vi "TEMPLATE_Constructor.vi"(8 "Error In":errorcluster) -> (0 "Error Out":errorcluster, 3 "OpaqueStruct Out":refnum<class "TEMPLATE_OpaqueStruct.lvclass">)   [LabVIEW 2013, in "Template.lvlib" / "TEMPLATE_OpaqueStruct.lvclass"]
uses:
  TEMPLATE_OpaqueStruct.lvclass
  TEMPLATE_OpaqueStruct.lvclass/TEMPLATE_OpaqueStruct.ctl
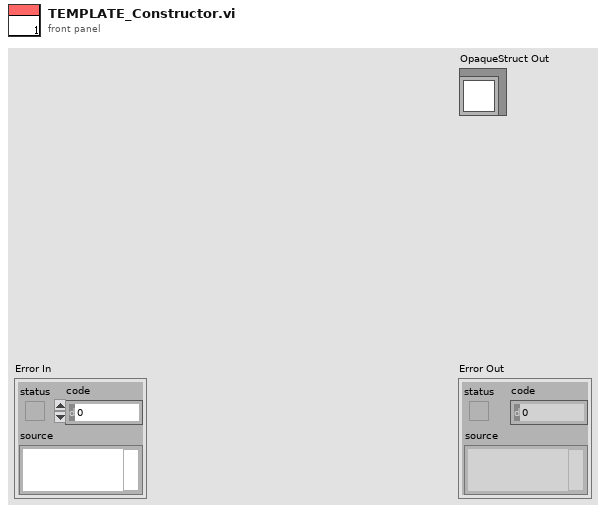
[diagram p1: front panel]
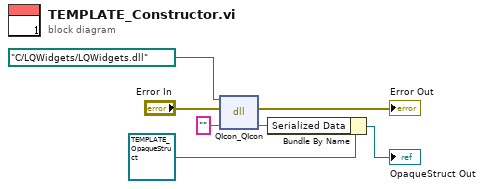
[diagram p0: block diagram]
diagram:
  n1 = dll-call lib="?" fn="QIcon_QIcon"(path in=path "C:/LQWidgets/LQWidgets.dll", error in="Error In", "obj"="") -> (error out=→"Error Out":errorcluster, "obj"=w3:string)  [unwired: 2 in, 1 out]
  n2 = Bundle By Name(cluster=refnum<class "TEMPLATE_OpaqueStruct.lvclass"> refnum ("QObject"), "Serialized Data"=w3) -> (→"OpaqueStruct Out":refnum<class "TEMPLATE_OpaqueStruct.lvclass">)
